vi "Auto Rotate.vi"(7 "RotateSpeed":dbl, 8 "Center":bool, 9 "RotateRight":bool, 10 "RotateLeft":bool, 11 "Gyroscope":dbl) -> (3 "Rotation Speed":dbl)   [LabVIEW 2014]
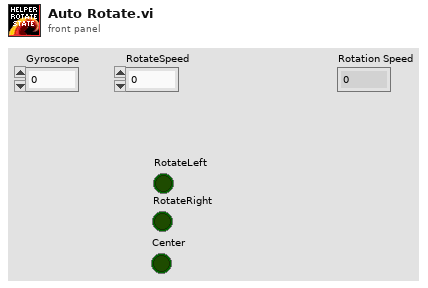
[diagram p1: front panel]
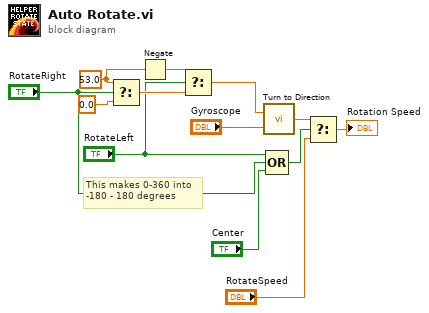
[diagram p0: block diagram]
diagram:
  w2 = 53.0
  # "This makes 0-360 into\n-180 - 180 degrees"
  n1 = Select(t=w2, s="RotateRight", f=0.0) -> (s? t:f=w12:dbl)
  n2 = Negate(x=w2) -> (-x=w1:dbl)
  n3 = Select(t=w1, s="RotateLeft", f=w12) -> (s? t:f=w4:dbl)
  n4 = call "Turn to Direction.vi"("Gyroscope"="Gyroscope", "Set"=w4) -> ("Rotation Speed"=w3:dbl)
  n5 = Compound Arithmetic op=OR("RotateLeft", "RotateRight", "Center") -> (w8:bool)
  n6 = Select(t=w3, s=w8, f="RotateSpeed") -> (s? t:f=→"Rotation Speed":dbl)
